vi "PWM_Lenkung.vi"(0 "vorne rechts":dbl=75.31181382488626, 1 "vorne links":dbl=29.917677039556622, 2 "Schräg rechts":dbl, 4 "Schräg links":dbl=31.586166184242515, 5 "PID gains out 2":T1={"proportional gain (Kc)"=0.5, "integral time (Ti, min)"=0.0, "derivative time (Td, min)"=0.002} {"proportional gain (Kc)" format="%#_10g"; "integral time (Ti, min)" format="%#_10g"; "derivative time (Td, min)" format="%#_10g"}) -> (14 "PWM Lenkung":dbl=0.3577035044911076)   [LabVIEW 2016]
doc: "PID Regelung für Servowert\n05.04.17_Tloe"
uses:
  <vilib>/addons/control/pid/pid.llb/PID (DBL).vi
  <vilib>/addons/control/pid/NI_PID_pid.lvlib
panel:
  in  "reinitialize? (F)":bool
  in  "y":dbl=20.0 format="%#_13g"
  in  "x":dbl=0.9
  # "vorher 0,9"
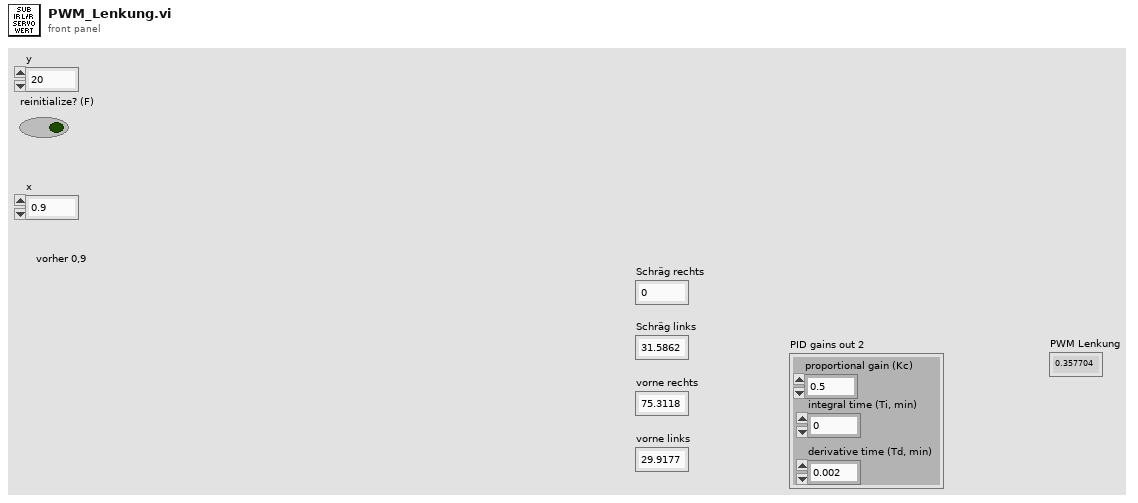
[diagram p1: front panel]
types:
  T1 = cluster{"proportional gain (Kc)":dbl, "integral time (Ti, min)":dbl, "derivative time (Td, min)":dbl}
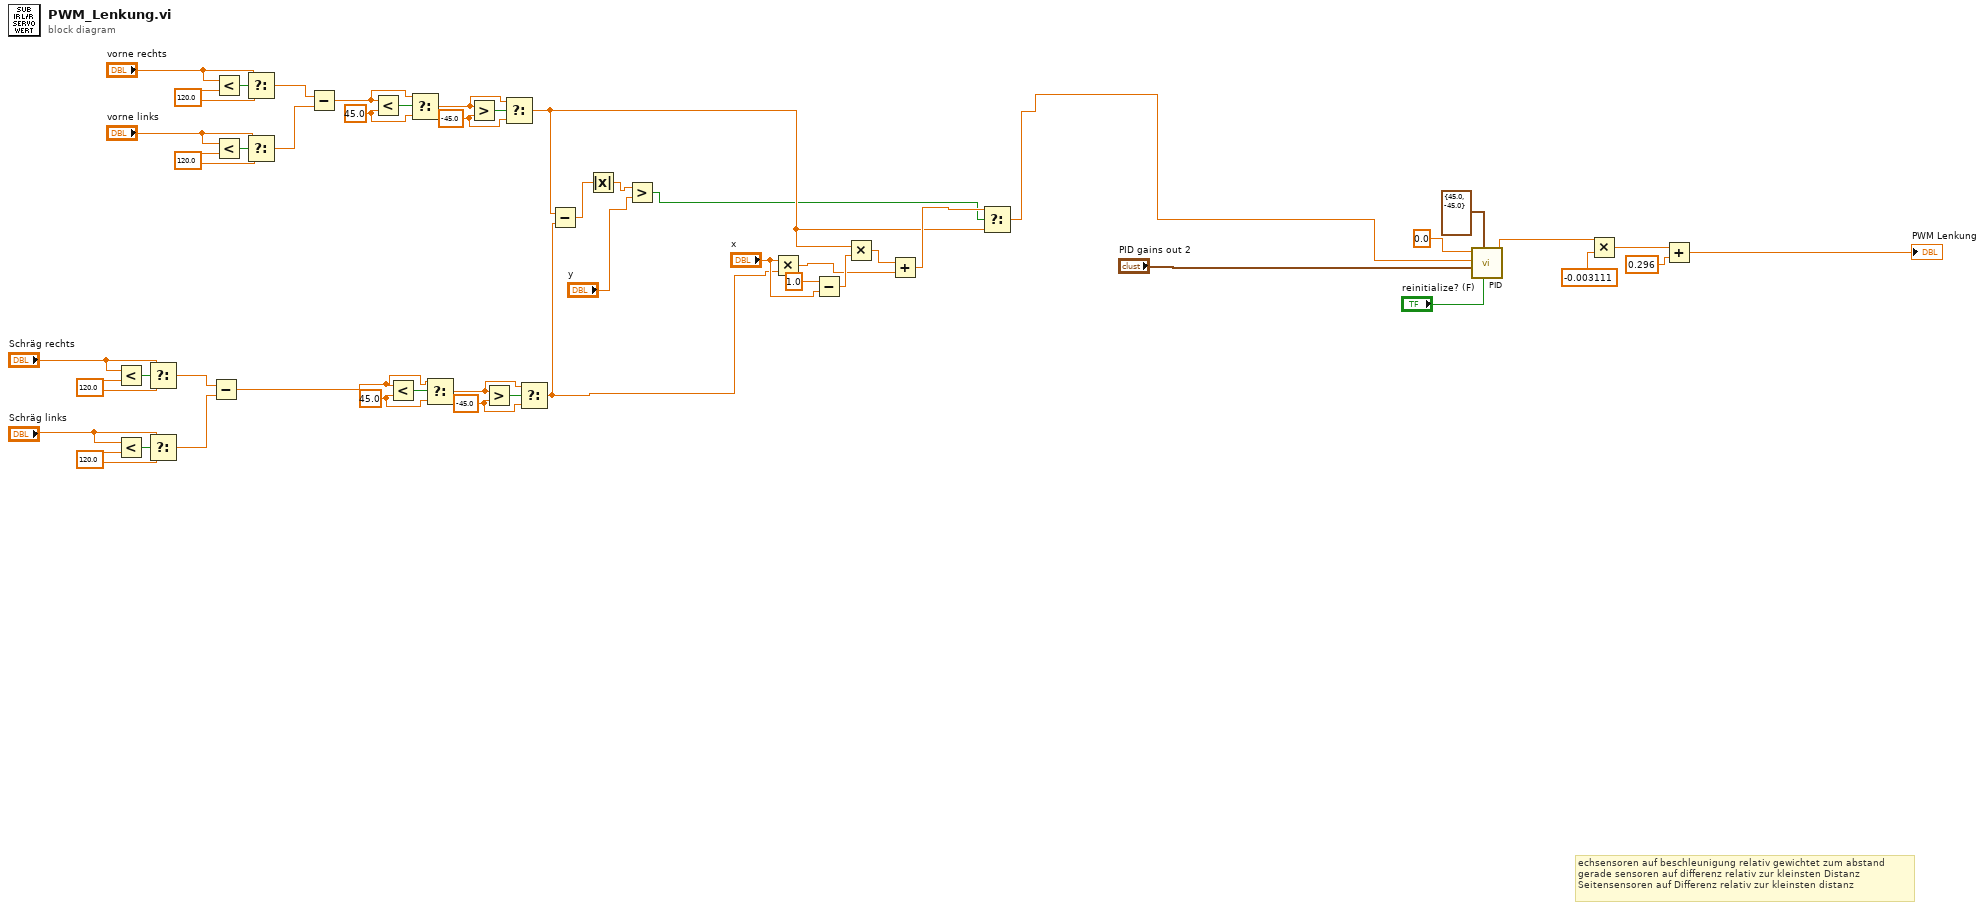
[diagram p0: block diagram]
diagram:
  w20 = 120.0 ("y")
  w24 = 120.0 ("y")
  w28 = 120.0 ("y")
  w31 = 120.0 ("y")
  w34 = -45.0 ("y")
  w37 = 45.0 ("y")
  w39 = -45.0 ("y")
  w42 = 45.0 ("y")
  # "echsensoren auf beschleunigung relativ gewichtet zum abstand\ngerade sensoren auf differenz relativ zur kleinsten Distanz\nSeitensensoren auf Differenz relativ zur kleinsten distanz"
  n1 = Less?(x="Schräg rechts", y=w24) -> (x < y?=w25:bool)
  n2 = Less?(x="Schräg links", y=w20) -> (x < y?=w21:bool)
  n3 = Select(t="Schräg rechts", s=w25, f=w24) -> (s? t:f=w23:dbl)
  n4 = Select(t="Schräg links", s=w21, f=w20) -> (s? t:f=w19:dbl)
  n5 = Subtract(x=w23, y=w19) -> (x-y=w5:dbl)
  n6 = Less?(x="vorne rechts", y=w31) -> (x < y?=w33:bool)
  n7 = Less?(x="vorne links", y=w28) -> (x < y?=w29:bool)
  n8 = Select(t="vorne rechts", s=w33, f=w31) -> (s? t:f=w30:dbl)
  n9 = Select(t="vorne links", s=w29, f=w28) -> (s? t:f=w26:dbl)
  n10 = Subtract(x=w30, y=w26) -> (x-y=w43:dbl)
  n11 = Less?(x=w43, y=w42) -> (x < y?=w44:bool)
  n12 = Less?(x=w5, y=w37) -> (x < y?=w38:bool)
  n13 = Select(t=w43, s=w44, f=w42) -> (s? t:f=w40:dbl)
  n14 = Select(t=w5, s=w38, f=w37) -> (s? t:f=w35:dbl)
  n15 = Greater?(x=w40, y=w39) -> (0:w41:bool)
  n16 = Greater?(x=w35, y=w34) -> (0:w36:bool)
  n17 = Select(t=w40, s=w41, f=w39) -> (s? t:f=w6:dbl)
  n18 = Select(t=w35, s=w36, f=w34) -> (s? t:f=w9:dbl)
  n19 = Subtract(x=w6, y=w9) -> (x-y=w3:dbl)
  n20 = Absolute Value(x=w3) -> (abs(x)=w2:dbl)
  n21 = Greater?(x=w2, y="y") -> (0:w4:bool)
  n22 = Multiply(x="x", y=w9) -> (x*y=w13:dbl)
  n23 = Subtract(x=1.0, y="x") -> (x-y=w16:dbl)
  n24 = Multiply(x=w6, y=w16) -> (x*y=w17:dbl)
  n25 = Add(x=w17, y=w13) -> (x+y=w10:dbl)
  n26 = Select(t=w10, s=w4, f=w6) -> (s? t:f=w1:dbl)
  n27 = call-poly <vilib>:"PID.vi"("reinitialize? (F)"="reinitialize? (F)", "output range"=cluster{"output high":dbl, "output low":dbl} {"output high"=45.0, "output low"=-45.0}, "PID gains"="PID gains out 2", "process variable"=w1, "setpoint"=0.0) -> ("output"=w50:dbl)  [unwired: 5 in, 1 out]
  n28 = Multiply(x=w50, y=-0.003111) -> (x*y=w47:dbl)
  n29 = Add(x=w47, y=0.296) -> (x+y=→"PWM Lenkung":dbl)
